vi "Generate UID.vi"(8 "Error In":errorcluster) -> (0 "error out":errorcluster, 3 "GUID":string)   [LabVIEW 2016, in "StringIntelliSense.lvlib" / "IntelliSenseStringControl.lvclass"]
uses:
  IntelliSenseStringControl.lvclass
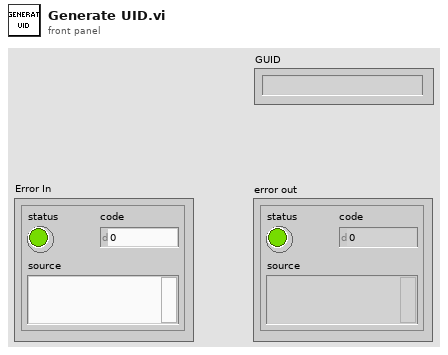
[diagram p1: front panel]
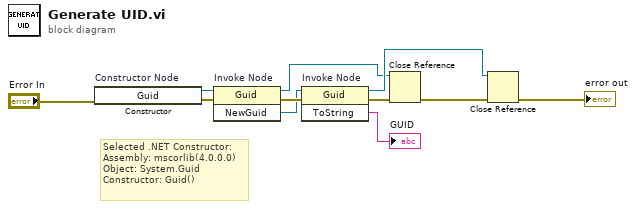
[diagram p0: block diagram]
diagram:
  # "Selected .NET Constructor:\nAssembly: mscorlib(4.0.0.0)\nObject: System.Guid\nConstructor: Guid()"
  n1 = constructor on="Constructor Node" class="System.Guid"(error in="Error In") -> (reference out=w2:refnum<k24>, error out=w3:errorcluster)  [unwired: 2 in, 1 out]
  n2 = invoke on="Invoke Node" class="Guid" method="NewGuid"(reference=w2, error in=w3) -> (reference out=w8:refnum<k24>, error out=w5:errorcluster, "NewGuid"=w4:refnum<k24>)  [unwired: 1 in]
  n3 = invoke on="Invoke Node" class="Guid" method="ToString"(reference=w4, error in=w5) -> (reference out=w9:refnum<k24>, error out=w6:errorcluster, "ToString"=→"GUID":string)  [unwired: 1 in]
  n4 = Close Reference(reference=w8, error in (no error)=w6) -> (error out=w7:errorcluster)
  n5 = Close Reference(reference=w9, error in (no error)=w7) -> (error out=→"error out":errorcluster)
